vi "OPC_server_param.vi"(11 "Regs":string[](array[string])) -> (3 "Parameters":T1[](array[typedef])=[{"name"="AI.AI", "data type"=111, "access level"=enum."read-only", "description"="AI Value Array", "period"=enum."500 ms"}, {"name"="AI.AI_ALRState", "data type"=106, "access level"=enum."read-only", "description"="AI ALR State Array", "period"=enum."500 ms"}, {"name"="AI.AI_Descriptions", "data type"=112, "access level"=enum."read-only", "description"="AI Descriptions Array", "period"=enum."on_load"}, {"name"="AI.AI_Names", "data type"=112, "access level"=enum."read-only", "description"="AI Names Array", "period"=enum."500 ms"}, {"name"="AI.AI_State", "data type"=106, "access level"=enum."read-only", "description"="AI State Array", "period"=enum."500 ms"}, {"name"="ALR.ALR", "data type"=101, "access level"=enum."read-only", "description"="ALARM Array", "period"=enum."100 ms"}, {"name"="ALR.ALR_Block", "data type"=101, "access level"=enum."read-only", "description"="ALR Blocked Array", "period"=enum."100 ms"}, {"name"="ALR.ALR_Descriptions", "data type"=112, "access level"=enum."read-only", "description"="ALR Descriptions Array", "period"=enum."on_load"}, {"name"="ALR.ALR_Names", "data type"=112, "access level"=enum."read-only", "description"="ALR Names Array", "period"=enum."100 ms"}, {"name"="ALR.ALR_Pcode", "data type"=112, "access level"=enum."read-only", "description"="ALR Param Names Array", "period"=enum."on_load"}, {"name"="ALR.ALR_State", "data type"=106, "access level"=enum."read-only", "description"="ALR State Array", "period"=enum."100 ms"}, {"name"="AO.AO", "data type"=111, "access level"=enum."read-only", "description"="AO Value Array", "period"=enum."500 ms"}, {"name"="AO.AO_ALRState", "data type"=106, "access level"=enum."read-only", "description"="AO ALR State Array", "period"=enum."500 ms"}, {"name"="AO.AO_Descriptions", "data type"=112, "access level"=enum."read-only", "description"="AO Descriptions Array", "period"=enum."on_load"}, {"name"="AO.AO_Names", "data type"=112, "access level"=enum."read-only", "description"="AO Names Array", "period"=enum."500 ms"}, {"name"="AO.AO_State", "data type"=106, "access level"=enum."read-only", "description"="AO State Array", "period"=enum."500 ms"}, {"name"="DI.DI", "data type"=101, "access level"=enum."read-only", "description"="DI Value Array", "period"=enum."100 ms"}, {"name"="DI.DI_ALRState", "data type"=106, "access level"=enum."read-only", "description"="DI ALR State Array", "period"=enum."100 ms"}, {"name"="DI.DI_Descriptions", "data type"=112, "access level"=enum."read-only", "description"="DI Descriptions Array", "period"=enum."on_load"}, {"name"="DI.DI_Names", "data type"=112, "access level"=enum."read-only", "description"="DI Names Array", "period"=enum."100 ms"}, {"name"="DI.DI_State", "data type"=106, "access level"=enum."read-only", "description"="DI State Array", "period"=enum."100 ms"}, {"name"="DO.DO", "data type"=101, "access level"=enum."read-only", "description"="DO Value Array", "period"=enum."100 ms"}, {"name"="DO.DO_ALRState", "data type"=106, "access level"=enum."read-only", "description"="DO ALR State Array", "period"=enum."100 ms"}, {"name"="DO.DO_Descriptions", "data type"=112, "access level"=enum."read-only", "description"="DO Descriptions Array", "period"=enum."on_load"}, {"name"="DO.DO_Names", "data type"=112, "access level"=enum."read-only", "description"="DO Names Array", "period"=enum."100 ms"}, {"name"="DO.DO_State", "data type"=106, "access level"=enum."read-only", "description"="DO State Array", "period"=enum."100 ms"}, {"name"="HT1.control", "data type"=12, "access level"=enum."none", "description"="HT1 reg input", "period"=enum."100 ms"}, {"name"="HT1.state", "data type"=12, "access level"=enum."read-only", "description"="HT1 reg output", "period"=enum."100 ms"}, {"name"="HT2.control", "data type"=12, "access level"=enum."none", "description"="HT2 reg input", "period"=enum."100 ms"}, {"name"="HT2.state", "data type"=12, "access level"=enum."read-only", "description"="HT2 reg output", "period"=enum."100 ms"}] {"data type" items=["Boolean"=1, "SByte"=2, "Byte"=3, "Int16"=4, "UInt16"=5, "Int32"=6, "UInt32"=7, "Int64"=8, "UInt64"=9, "Float"=10, "Double"=11, "String"=12, "DateTime"=13, "ByteString"=15, "Array of Boolean"=101, "Array of SByte"=102, "Array of Byte"=103, "Array of Int16"=104, "Array of UInt16"=105, "Array of Int32"=106, "Array of UInt32"=107, "Array of Int64"=108, "Array of UInt64"=109, "Array of Float"=110, "Array of Double"=111, "Array of String"=112, "Array of DateTime"=113, "Array of ByteString"=115, "Matrix of Boolean"=201, "Matrix of SByte"=202, "Matrix of Byte"=203, "Matrix of Int16"=204, "Matrix of UInt16"=205, "Matrix of Int32"=206, "Matrix of UInt32"=207, "Matrix of Int64"=208, "Matrix of UInt64"=209, "Matrix of Float"=210, "Matrix of Double"=211, "Matrix of String "=212, "Matrix of DateTime"=213, "Matrix of ByteString"=215]})   [LabVIEW 2021, in "Param_h0gm1.lvlib"]
uses:
  Param_h0gm1.lvlib
  OPC/OPC tag.ctl
  <vilib>/OPCUA/controls/Data Type.ctl
  OPC/Access level.ctl
  OPC/Period.ctl
  OPC/OPC addons.lvlib
panel:
  in  "OPC Param unsorted":T1[](array[typedef])=[{"name"="AI.AI", "data type"=111, "access level"=enum."read-only", "description"="AI Value Array", "period"=enum."500 ms"}, {"name"="AI.AI_State", "data type"=106, "access level"=enum."read-only", "description"="AI State Array", "period"=enum."500 ms"}, {"name"="AI.AI_ALRState", "data type"=106, "access level"=enum."read-only", "description"="AI ALR State Array", "period"=enum."500 ms"}, {"name"="AI.AI_Names", "data type"=112, "access level"=enum."read-only", "description"="AI Names Array", "period"=enum."500 ms"}, {"name"="AI.AI_Descriptions", "data type"=115, "access level"=enum."read-only", "description"="AI Descriptions Array", "period"=enum."on_load"}, {"name"="DI.DI", "data type"=101, "access level"=enum."read-only", "description"="DI Value Array", "period"=enum."100 ms"}, {"name"="DI.DI_State", "data type"=106, "access level"=enum."read-only", "description"="DI State Array", "period"=enum."100 ms"}, {"name"="DI.DI_ALRState", "data type"=106, "access level"=enum."read-only", "description"="DI ALR State Array", "period"=enum."100 ms"}, {"name"="DI.DI_Names", "data type"=112, "access level"=enum."read-only", "description"="DI Names Array", "period"=enum."100 ms"}, {"name"="DI.DI_Descriptions", "data type"=115, "access level"=enum."read-only", "description"="DI Descriptions Array", "period"=enum."on_load"}, {"name"="AO.AO", "data type"=111, "access level"=enum."read-only", "description"="AO Value Array", "period"=enum."500 ms"}, {"name"="AO.AO_State", "data type"=106, "access level"=enum."read-only", "description"="AO State Array", "period"=enum."1 s"}, {"name"="AO.AO_ALRState", "data type"=106, "access level"=enum."read-only", "description"="AO ALR State Array", "period"=enum."1 s"}, {"name"="AO.AO_Names", "data type"=112, "access level"=enum."read-only", "description"="AO Names Array", "period"=enum."500 ms"}, {"name"="AO.AO_Descriptions", "data type"=115, "access level"=enum."read-only", "description"="AO Descriptions Array", "period"=enum."on_load"}, {"name"="DO.DO", "data type"=101, "access level"=enum."read-only", "description"="DO Value Array", "period"=enum."100 ms"}, {"name"="DO.DO_State", "data type"=106, "access level"=enum."read-only", "description"="DO State Array", "period"=enum."1 s"}, {"name"="DO.DO_ALRState", "data type"=106, "access level"=enum."read-only", "description"="DO ALR State Array", "period"=enum."1 s"}, {"name"="DO.DO_Names", "data type"=112, "access level"=enum."read-only", "description"="DO Names Array", "period"=enum."100 ms"}, {"name"="DO.DO_Descriptions", "data type"=115, "access level"=enum."read-only", "description"="DO Descriptions Array", "period"=enum."on_load"}, {"name"="ALR.ALR_blocked", "data type"=101, "access level"=enum."read-only", "description"="ALR Blocked Array", "period"=enum."500 ms"}, {"name"="ALR.ALR_ON", "data type"=101, "access level"=enum."read-only", "description"="ALR ON Array", "period"=enum."500 ms"}, {"name"="ALR.t_ms", "data type"=107, "access level"=enum."read-only", "description"="ALR t Array", "period"=enum."500 ms"}, {"name"="ALR.ack_state", "data type"=107, "access level"=enum."read-only", "description"="ALR State Array", "period"=enum."500 ms"}, {"name"="ALR.color", "data type"=107, "access level"=enum."read-only", "description"="AI Value Array", "period"=enum."500 ms"}, {"name"="ALR.ALR_Names", "data type"=112, "access level"=enum."read-only", "description"="ALR Names Array", "period"=enum."500 ms"}, {"name"="ALR.ALR_Descriptions", "data type"=115, "access level"=enum."read-only", "description"="ALR Descriptions Array", "period"=enum."on_load"}, {"name"="ALR.ALR_Pcode", "data type"=115, "access level"=enum."read-only", "description"="ALR Param Names Array", "period"=enum."on_load"}, {"name"="CONTROL.control", "data type"=12, "access level"=enum."write-only", "description"="Control channel", "period"=enum."100 ms"}] {"data type" items=["Boolean"=1, "SByte"=2, "Byte"=3, "Int16"=4, "UInt16"=5, "Int32"=6, "UInt32"=7, "Int64"=8, "UInt64"=9, "Float"=10, "Double"=11, "String"=12, "DateTime"=13, "ByteString"=15, "Array of Boolean"=101, "Array of SByte"=102, "Array of Byte"=103, "Array of Int16"=104, "Array of UInt16"=105, "Array of Int32"=106, "Array of UInt32"=107, "Array of Int64"=108, "Array of UInt64"=109, "Array of Float"=110, "Array of Double"=111, "Array of String"=112, "Array of DateTime"=113, "Array of ByteString"=115, "Matrix of Boolean"=201, "Matrix of SByte"=202, "Matrix of Byte"=203, "Matrix of Int16"=204, "Matrix of UInt16"=205, "Matrix of Int32"=206, "Matrix of UInt32"=207, "Matrix of Int64"=208, "Matrix of UInt64"=209, "Matrix of Float"=210, "Matrix of Double"=211, "Matrix of String "=212, "Matrix of DateTime"=213, "Matrix of ByteString"=215]}
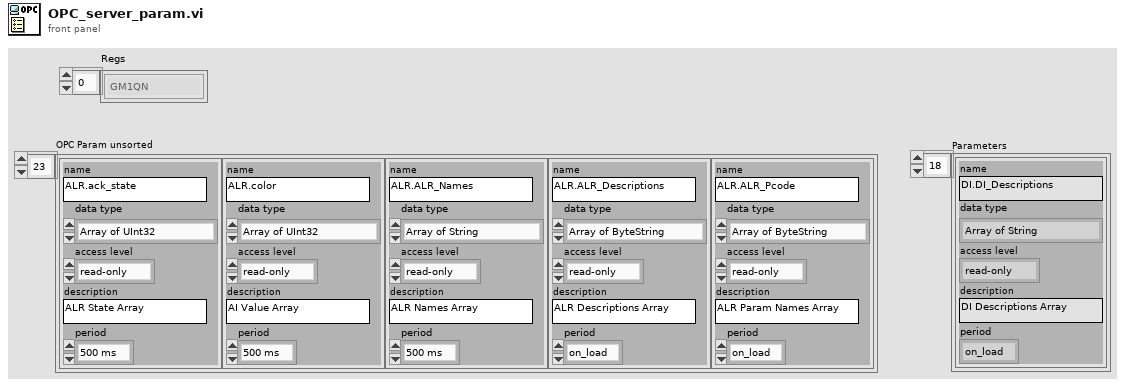
[diagram p1: front panel]
types:
  T1 = typedef "OPC addons.lvlib/OPC tag.ctl" = cluster{"name":string, "data type":T2, "access level":T3, "description":string, "period":T4}
  T2 = typedef "Data Type.ctl" = u16
  T3 = typedef "OPC addons.lvlib/Access level.ctl" = enum16{"none", "read-only", "write-only", "read/write"}
  T4 = typedef "OPC addons.lvlib/Period.ctl" = enum16{"on_load", "100 ms", "500 ms", "1 s"}
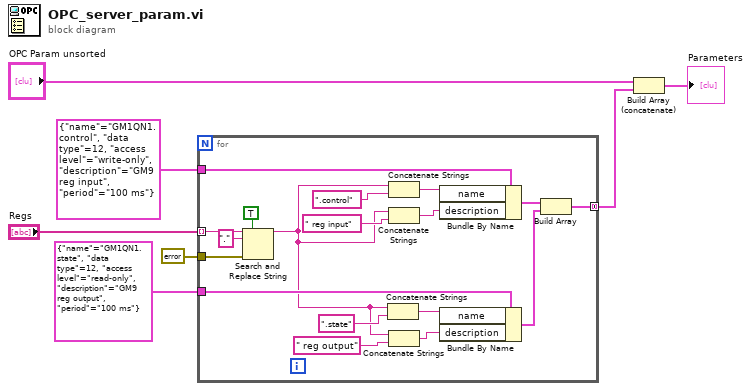
[diagram p0: block diagram]
diagram:
  n1 = for {
    tunnel: T1 {"name"="GM1QN1.control", "data type"=12, "access level"=enum."write-only", "description"="GM9 reg input", "period"=enum."100 ms"} ("AI") -> [w25]
    tunnel: T1 {"name"="GM1QN1.state", "data type"=12, "access level"=enum."read-only", "description"="GM9 reg output", "period"=enum."100 ms"} ("AI") -> [w20]
    tunnel: [w13] -> w1 mode=concatenating
    tunnel: "Regs" -> [w10] mode=indexing
    tunnel: errorcluster {"status"=FALSE, "code"=0, "source"=""} ("error in (no error)") -> [w8]
    n2 = Search and Replace String(replace all?=TRUE ("replace all? (F)"), input string=w10, search string=".", error in=w8) -> (result string=w11:string)  [unwired: 4 in, 3 out]
    n3 = Concatenate Strings(w11, ".state" ("string")) -> (w17:string)
    n4 = Concatenate Strings(w11, ".control" ("string")) -> (w23:string)
    n5 = Concatenate Strings(w11, " reg input" ("string")) -> (w21:string)
    n6 = Concatenate Strings(w11, " reg output" ("string")) -> (w16:string)
    n7 = Bundle By Name(cluster=w25, "name"=w23, "description"=w21) -> (w15:T1)
    n8 = Bundle By Name(cluster=w20, "name"=w17, "description"=w16) -> (w14:T1)
    n9 = Build Array(w15, w14) -> (w13:T1[])
  }
  n10 = Build Array (concatenate)("OPC Param unsorted", w1) -> (→"Parameters":T1[])
